vi "Stream LLP Packets from Disk.vi"(0 "fpga interface in":refnum<k20>, 1 "'stop' notifier":refnum<notifier>, 5 "serial output channel":string, 7 "llp data file path":path, 9 "maximum write size (elements)":u32=40960, 11 "error in (no error)":errorcluster, 12 "write timeout (s)":dbl=1.0) -> (4 "fpga interface out":refnum<k20>, 15 "error out":errorcluster)   [LabVIEW 2023, in "GettingStarted_Gen_148X_Host.lvlib"]
uses:
  GettingStarted_Gen_148X_Host.lvlib
  Types/148x_Gen_FPGA_Reference.ctl
  <vilib>/rvi/errors/niLvFpgaAdjustHostInterfaceError.vi
  <vilib>/rvi/interface/nirviMethod/nirviMethod.xnode
  <instrlib>/FlexRIO/Automotive Vision Utility/v1/Host/Automotive Vision Utility.lvlib
  <vilib>/rvi/errors/niLvFpgaMergeErrorWithErrorCode.vi
  <vilib>/FPGAPlugInAG/Dynamic/niLvFpga_AcquireWriteRegionFifo_Dynamic.vi
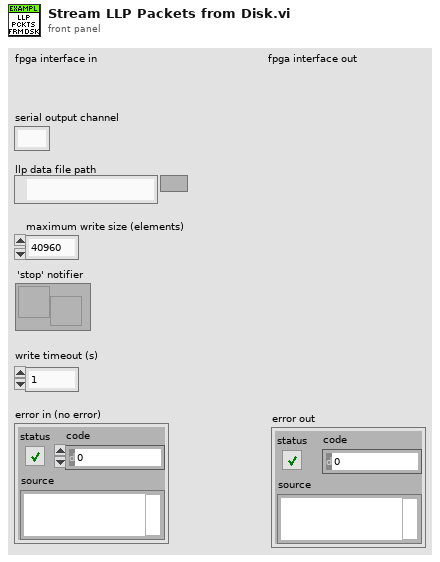
[diagram p1: front panel]
types:
  T1 = typedef "Automotive Vision Utility.lvlib/Serial Channel Type.ctl" = enum16{"Serial Input Channel", "Serial Output Channel", "Unknown Channel Type"}
  T2 = typedef "GettingStarted_Gen_148X_Host.lvlib/148x_Gen_FPGA_Reference.ctl" = refnum<k20>
  T3 = enum16{"open", "open or create", "create or replace", "create", "open (read-only)"}
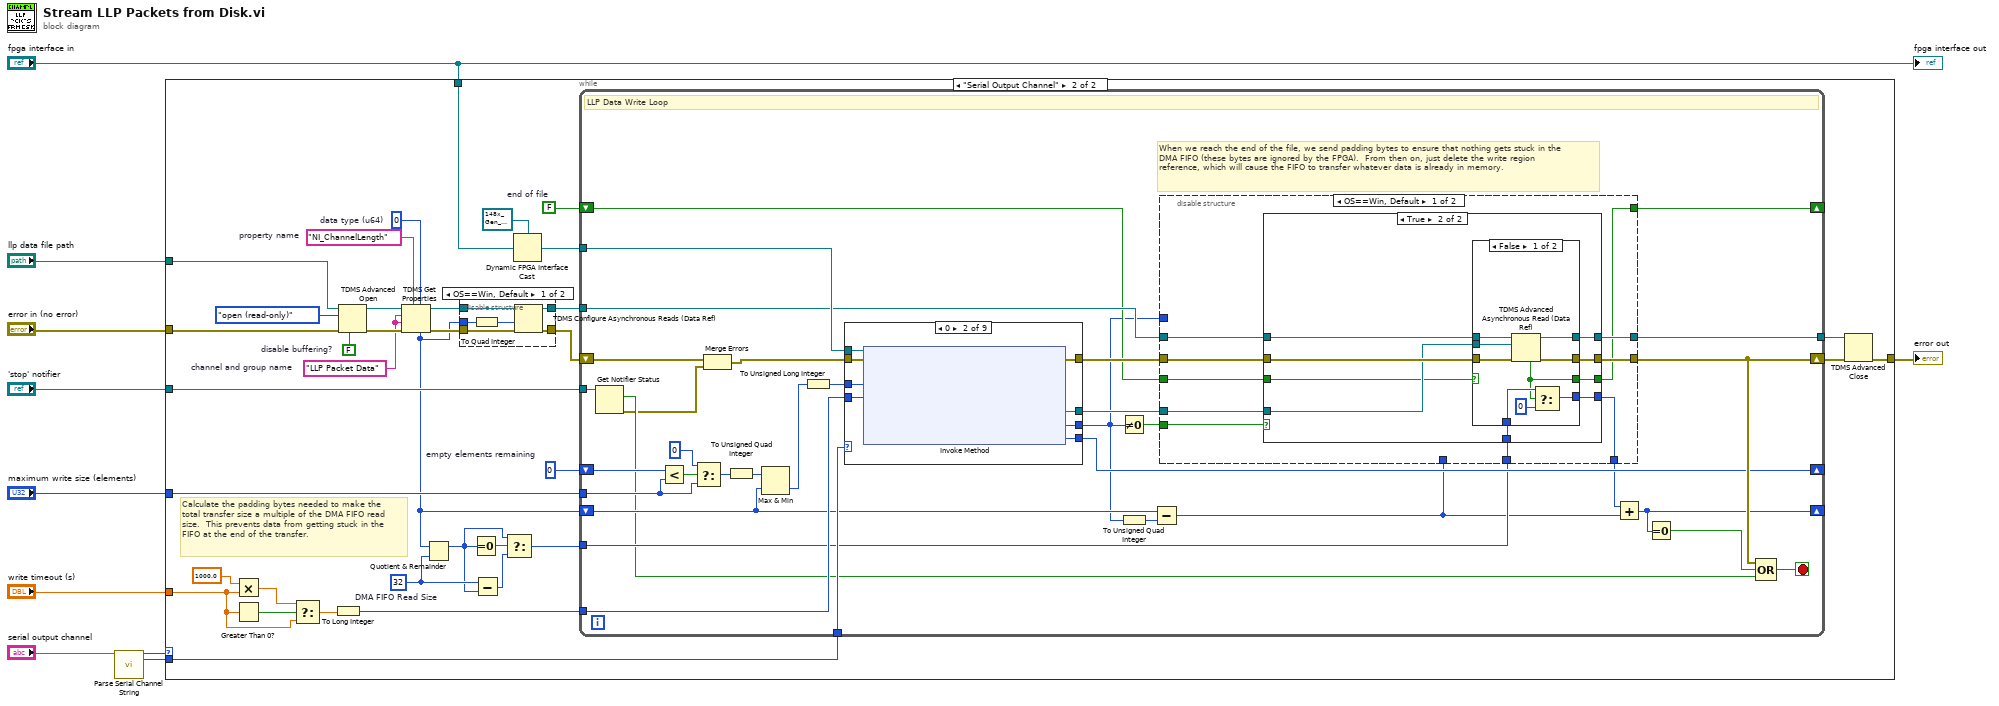
[diagram p0: block diagram]
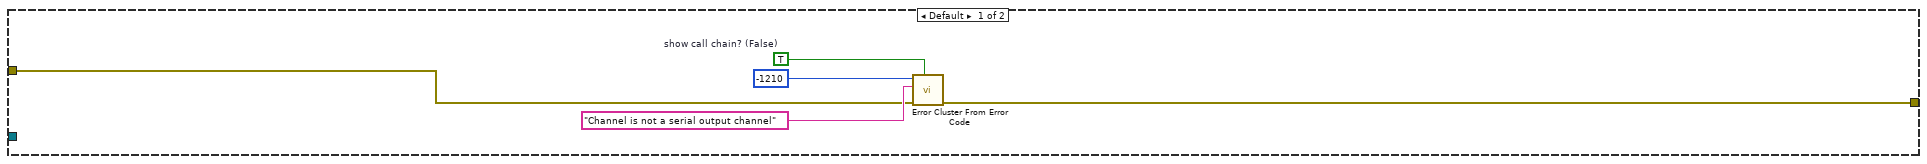
[diagram p2: hidden frame]
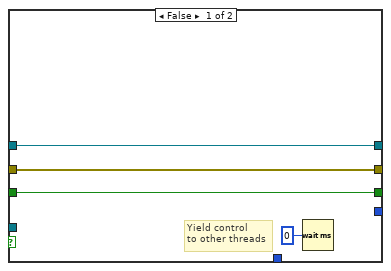
[diagram p3: hidden frame]
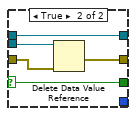
[diagram p4: hidden frame]
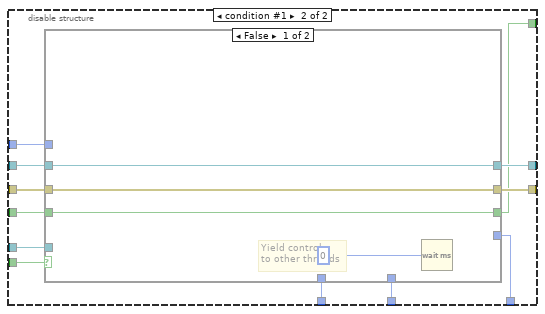
[diagram p5: hidden frame]
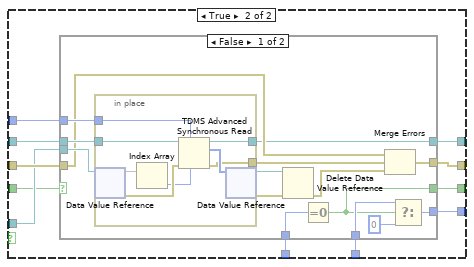
[diagram p6: hidden frame]
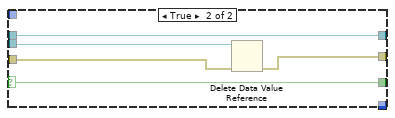
[diagram p7: hidden frame]
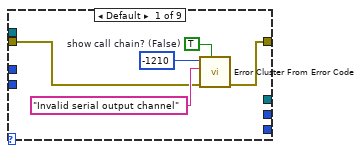
[diagram p8: hidden frame]
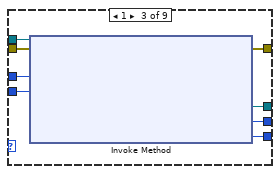
[diagram p9: hidden frame]
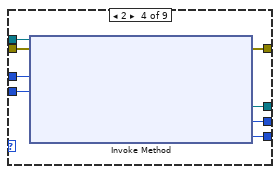
[diagram p10: hidden frame]
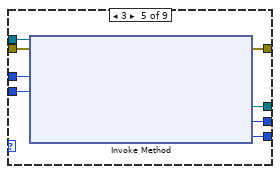
[diagram p11: hidden frame]
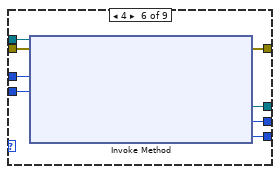
[diagram p12: hidden frame]
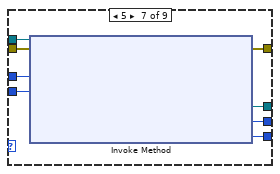
[diagram p13: hidden frame]
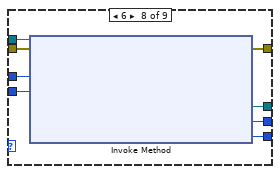
[diagram p14: hidden frame]
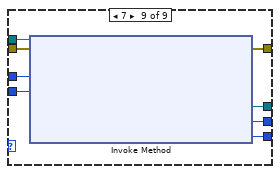
[diagram p15: hidden frame]
diagram:
  n1 = call <instrlib>:"Parse Serial Channel String.vi"("serial channel string"="serial output channel") -> ("serial channel type"=w6:T1, "channel number"=w7:i32)  [unwired: 13 in]
  n2 = case shown="\"Serial Output Channel\"" w6 {
    tunnel: "error in (no error)" -> [w13 w51]
    tunnel: [w12 w34] -> w9
    tunnel: "fpga interface in" -> [_ w47]
    tunnel: w7 -> [_ w44]
    tunnel: "maximum write size (elements)" -> [_ w43]
    tunnel: "llp data file path" -> [_ w41]
    tunnel: "write timeout (s)" -> [_ w28]
    tunnel: "'stop' notifier" -> [_ w37]
    frame Default {
      w11 = TRUE  # show call chain? (False)
      n3 = call <vilib>:"Error Cluster From Error Code.vi"("show call chain? (False)"=w11, "error in (no error)"=w13, "error message (\"\")"="Channel is not a serial output channel" ("error message (\"\")"), "error code (0)"=-1210) -> ("error out"=w12:errorcluster)  [unwired: 5 in]
    }
    frame "Serial Output Channel" {
      w25 = u64 32  # DMA FIFO Read Size
      w27 = u32 0  # empty elements remaining
      w33 = FALSE  # end of file
      w38 = u64 0  # data type (u64)
      w18 = "NI_ChannelLength"  # property name
      w49 = FALSE  # disable buffering?
      w35 = "LLP Packet Data"  # channel and group name
      # "Calculate the padding bytes needed to make the total transfer size a multiple of the DMA FIFO read size.  This prevents data from getting stuck in the FIFO at the end of the transfer."
      n4 = Multiply(x=1000.0 ("y"), y=w28) -> (x*y=w30:dbl)
      n5 = Greater Than 0?(x=w28) -> (x > 0?=w29:bool)
      n6 = Select(t=w30, s=w29, f=w28) -> (s? t:f=w31:dbl)
      n7 = To Long Integer(number=w31) -> (32bit integer=w36:i32)
      n8 = TDMS Advanced Open(6:w49, 8:w51, 10:T3."open (read-only)" ("operation (0:open)"), 11:w41) -> (0:w39:errorcluster, 3:w40:refnum<k34>)  [unwired: 1 in, 1 out]
      n9 = TDMS Get Properties(5:w38, 7:w18, 8:w39, 9:w35, 10:w35, 11:w40) -> (0:w19:errorcluster, 3:w20:refnum<k34>, 4:w17:u64)  [unwired: 3 out]
      n10 = Quotient & Remainder(x=w17, y=w25) -> (x-y*floor(x/y)=w23:u64)  [unwired: 1 out]
      n11 = disable-structure shown="OS==Win, Default" {
        disable-tunnel: w19 -> [w249 w254]
        disable-tunnel: [w251 w253] -> w22
        disable-tunnel: [w250 w254] -> w21
        disable-tunnel: w20 -> [w252 w253]
        disable-tunnel: w17 -> [w248 _]
        frame condition #0 (active) {
          n12 = To Quad Integer(1:w248) -> (0:w247:i64)
          n13 = TDMS Configure Asynchronous Reads (Data Ref)(8:w249, 9:w247, 11:w252) -> (0:w250:errorcluster, 3:w251:refnum<k34>)  [unwired: 2 in]
        }
        frame condition #1 {
        }
      }
      n14 = Equal To 0?(x=w23) -> (x = 0?=w26:bool)
      n15 = Subtract(x=w25, y=w23) -> (x-y=w24:u64)
      n16 = Select(t=w23, s=w26, f=w24) -> (s? t:f=w16:u64)
      n17 = Dynamic FPGA Interface Cast(Session In=T2 refnum ("FPGA VI Reference Out"), Type=w47) -> (Session Out=w46:T2)
      n18 = while {
        shift-right: [w77] -> w45
        shift-left: w21 -> [w53]
        tunnel: w46 -> [w78]
        shift-right: [w60] -> _
        shift-left: w17 -> [w64]
        tunnel: w22 -> [w73]
        tunnel: [w82] -> w42
        tunnel: w44 -> [w81]
        tunnel: w43 -> [w68]
        tunnel: w36 -> [w75]
        tunnel: w37 -> [w56]
        shift-right: [w72] -> _
        shift-left: w33 -> [w71]
        shift-right: [w70] -> _
        shift-left: w27 -> [w69]
        tunnel: w16 -> [w62]
        stop <- w85 stop-if-true
        # "When we reach the end of the file, we send padding bytes to ensure that nothing gets stuck in the DMA FIFO (these bytes are ignored by the FPGA).  From then on, just delete the write region reference, which will cause the FIFO to transfer whatever data is already in memory."
        # "LLP Data Write Loop"
        n19 = Get Notifier Status(notifier=w56) -> (current notification=w55:bool, error out=w52:errorcluster)  [unwired: 1 in, 3 out]
        n20 = Less?(x=w69, y=w68) -> (x < y?=w80:bool)
        n21 = Select(t=u32 0, s=w80, f=w68) -> (s? t:f=w66:u32)
        n22 = Merge Errors(w53, w52) -> (w54:errorcluster)
        n23 = To Unsigned Quad Integer(1:w66) -> (0:w65:u64)
        n24 = Max & Min(x=w65, y=w64) -> (min(x,y)=w63:u64)  [unwired: 1 out]
        n25 = To Unsigned Long Integer(number=w63) -> (unsigned 32bit integer=w58:u32)
        n26 = case shown="0" w81 {
          tunnel: w78 -> [_ w190 w198 w206 w214 w222 w230 w238 w246]
          tunnel: [_ w189 w197 w205 w213 w221 w229 w237 w245] -> w79
          tunnel: [_ w188 w196 w204 w212 w220 w228 w236 w244] -> w57
          tunnel: w58 -> [_ w187 w195 w203 w211 w219 w227 w235 w243]
          tunnel: [w180 w185 w193 w201 w209 w217 w225 w233 w241] -> w84
          tunnel: [_ w186 w194 w202 w210 w218 w226 w234 w242] -> w70
          tunnel: w54 -> [w178 w184 w192 w200 w208 w216 w224 w232 w240]
          tunnel: w75 -> [_ w183 w191 w199 w207 w215 w223 w231 w239]
          frame Default {
            w179 = TRUE  # show call chain? (False)
            n27 = call <vilib>:"Error Cluster From Error Code.vi"("show call chain? (False)"=w179, "error in (no error)"=w178, "error message (\"\")"="Invalid serial output channel" ("error message (\"\")"), "error code (0)"=-1210) -> ("error out"=w180:errorcluster)  [unwired: 5 in]
          }
          frame 0 {
            n28 = xnode "Invoke Method"("FPGA VI Reference In"=w190, "error in"=w184, "Number of Elements"=w187, "Timeout (ms)"=w183) -> ("error out"=w185:errorcluster, "Write Region Reference"=w189:refnum<data-value>, "Elements In Region"=w188:u32, "Empty Elements Remaining"=w186:u32)  [unwired: 1 out]
          }
          frame 1 {
            n29 = xnode "Invoke Method"("FPGA VI Reference In"=w198, "error in"=w192, "Number of Elements"=w195, "Timeout (ms)"=w191) -> ("error out"=w193:errorcluster, "Write Region Reference"=w197:refnum<data-value>, "Elements In Region"=w196:u32, "Empty Elements Remaining"=w194:u32)  [unwired: 1 out]
          }
          frame 2 {
            n30 = xnode "Invoke Method"("FPGA VI Reference In"=w206, "error in"=w200, "Number of Elements"=w203, "Timeout (ms)"=w199) -> ("error out"=w201:errorcluster, "Write Region Reference"=w205:refnum<data-value>, "Elements In Region"=w204:u32, "Empty Elements Remaining"=w202:u32)  [unwired: 1 out]
          }
          frame 3 {
            n31 = xnode "Invoke Method"("FPGA VI Reference In"=w214, "error in"=w208, "Number of Elements"=w211, "Timeout (ms)"=w207) -> ("error out"=w209:errorcluster, "Write Region Reference"=w213:refnum<data-value>, "Elements In Region"=w212:u32, "Empty Elements Remaining"=w210:u32)  [unwired: 1 out]
          }
          frame 4 {
            n32 = xnode "Invoke Method"("FPGA VI Reference In"=w222, "error in"=w216, "Number of Elements"=w219, "Timeout (ms)"=w215) -> ("error out"=w217:errorcluster, "Write Region Reference"=w221:refnum<data-value>, "Elements In Region"=w220:u32, "Empty Elements Remaining"=w218:u32)  [unwired: 1 out]
          }
          frame 5 {
            n33 = xnode "Invoke Method"("FPGA VI Reference In"=w230, "error in"=w224, "Number of Elements"=w227, "Timeout (ms)"=w223) -> ("error out"=w225:errorcluster, "Write Region Reference"=w229:refnum<data-value>, "Elements In Region"=w228:u32, "Empty Elements Remaining"=w226:u32)  [unwired: 1 out]
          }
          frame 6 {
            n34 = xnode "Invoke Method"("FPGA VI Reference In"=w238, "error in"=w232, "Number of Elements"=w235, "Timeout (ms)"=w231) -> ("error out"=w233:errorcluster, "Write Region Reference"=w237:refnum<data-value>, "Elements In Region"=w236:u32, "Empty Elements Remaining"=w234:u32)  [unwired: 1 out]
          }
          frame 7 {
            n35 = xnode "Invoke Method"("FPGA VI Reference In"=w246, "error in"=w240, "Number of Elements"=w243, "Timeout (ms)"=w239) -> ("error out"=w241:errorcluster, "Write Region Reference"=w245:refnum<data-value>, "Elements In Region"=w244:u32, "Empty Elements Remaining"=w242:u32)  [unwired: 1 out]
          }
        }
        n36 = Not Equal To 0?(x=w57) -> (x != 0?=w83:bool)
        n37 = To Unsigned Quad Integer(1:w57) -> (0:w76:u64)
        n38 = Subtract(x=w64, y=w76) -> (x-y=w59:u64)
        n39 = disable-structure shown="OS==Win, Default" {
          disable-tunnel: w84 -> [w95 w134]
          disable-tunnel: w83 -> [w94 w133]
          disable-tunnel: [w93 w132] -> w82
          disable-tunnel: w79 -> [w92 w131]
          disable-tunnel: [w91 w130] -> w77
          disable-tunnel: w73 -> [w90 w129]
          disable-tunnel: [w89 w128] -> w72
          disable-tunnel: w71 -> [w88 w127]
          disable-tunnel: w57 -> [_ w126]
          disable-tunnel: w62 -> [w87 w124]
          disable-tunnel: [w86 w125] -> w61
          disable-tunnel: w59 -> [_ w123]
          frame condition #0 (active) {
            n40 = case shown="True" w94 {
              tunnel: w90 -> [w99 w105]
              tunnel: [w99 w108] -> w93
              tunnel: w95 -> [w98 w106]
              tunnel: [w98 w107] -> w91
              tunnel: w92 -> [_ w104]
              tunnel: [w96 w103] -> w89
              tunnel: w88 -> [w96 w102]
              tunnel: w87 -> [_ w101]
              tunnel: [_ w100] -> w86
              frame False {
                # "Yield control\nto other threads"
                n41 = Wait (ms)(milliseconds to wait=u32 0) -> ()  [unwired: 1 out]
              }
              frame True {
                n42 = case shown="False" w102 {
                  selector: w102 -> [_ w118]
                  tunnel: [w117 w122] -> w108
                  tunnel: [w116 w119] -> w107
                  tunnel: w106 -> [w115 w120]
                  tunnel: w105 -> [w114 w122]
                  tunnel: w104 -> [w113 w121]
                  tunnel: [w110 w118] -> w103
                  tunnel: w101 -> [w111 _]
                  tunnel: [w109 _] -> w100
                  frame False {
                    n43 = TDMS Advanced Asynchronous Read (Data Ref)(8:w115, 10:w113, 11:w114) -> (0:w116:errorcluster, 3:w117:refnum<k34>, 4:w110:bool)  [unwired: 1 in]
                    n44 = Select(t=w111, s=w110, f=u64 0) -> (s? t:f=w109:u64)
                  }
                  frame True {
                    n45 = Delete Data Value Reference(data value reference=w121, error in=w120) -> (error out=w119:errorcluster)  [unwired: 1 out]
                  }
                }
              }
            }
          }
          frame condition #1 {
            n46 = case shown="False" w133 {
              tunnel: w129 -> [w138 w146]
              tunnel: [w138 w149] -> w132
              tunnel: w134 -> [w137 w147]
              tunnel: [w137 w148] -> w130
              tunnel: w131 -> [_ w145]
              tunnel: [w135 w144] -> w128
              tunnel: w127 -> [w135 w143]
              tunnel: w126 -> [_ w142]
              tunnel: [_ w141] -> w125
              tunnel: w124 -> [_ w140]
              tunnel: w123 -> [_ w139]
              frame False {
                # "Yield control\nto other threads"
                n47 = Wait (ms)(milliseconds to wait=u32 0) -> ()  [unwired: 1 out]
              }
              frame True {
                n48 = case shown="False" w143 {
                  selector: w143 -> [_ w173]
                  tunnel: [w155 w177] -> w149
                  tunnel: [w159 w174] -> w148
                  tunnel: w147 -> [w156 w175]
                  tunnel: w146 -> [w162 w177]
                  tunnel: w145 -> [w164 w176]
                  tunnel: [w151 w173] -> w144
                  tunnel: w142 -> [w163 _]
                  tunnel: [w153 _] -> w141
                  tunnel: w140 -> [w152 _]
                  tunnel: w139 -> [w150 _]
                  frame False {
                    n49 = in-place {
                      in-place-border: w163 -> [w172]
                      in-place-border: w162 -> [w170]
                      in-place-border: [w166] -> w157
                      in-place-border: [w165] -> w155
                      n50 = in-place-dvr #1(w164) -> (w169:u8[], w171:errorcluster)
                      n51 = Index Array(array=w169) -> (element=w168:u8)  [unwired: 1 in]
                      n52 = TDMS Advanced Synchronous Read(6:w168, 7:w172, 8:w171, 11:w170) -> (0:w166:errorcluster, 2:w167:u8[], 3:w165:refnum<k34>)  [unwired: 1 out]
                      n53 = in-place-dvr #1(w167) -> (w160:refnum<data-value>, w161:errorcluster)
                    }
                    n54 = Delete Data Value Reference(data value reference=w160, error in=w161) -> (error out=w158:errorcluster)  [unwired: 1 out]
                    n55 = Equal To 0?(x=w150) -> (x = 0?=w151:bool)
                    n56 = Merge Errors(w156, w157, w158) -> (w159:errorcluster)
                    n57 = Select(t=w152, s=w151, f=u64 0) -> (s? t:f=w153:u64)
                  }
                  frame True {
                    n58 = Delete Data Value Reference(data value reference=w176, error in=w175) -> (error out=w174:errorcluster)  [unwired: 1 out]
                  }
                }
              }
            }
          }
        }
        n59 = Add(x=w61, y=w59) -> (x+y=w60:u64)
        n60 = Equal To 0?(x=w60) -> (x = 0?=w74:bool)
        n61 = Compound Arithmetic op=OR(w77, w74, w55) -> (w85:bool)
      }
      n62 = TDMS Advanced Close(8:w45, 11:w42) -> (0:w34:errorcluster)  [unwired: 2 in, 1 out]
    }
  }
  "error out" <- w9
  "fpga interface out" <- "fpga interface in"
